vi "As PropertyObject.vi"(8 "error in (no error)":errorcluster, 11 "Execution in":refnum<class "Execution.lvclass">) -> (0 "error out":errorcluster, 2 "PropertyObject":refnum<k7>, 3 "Execution out":refnum<class "Execution.lvclass">)   [LabVIEW 2020, in "TSnax.lvlib" / "Execution.lvclass"]
uses:
  Execution.lvclass
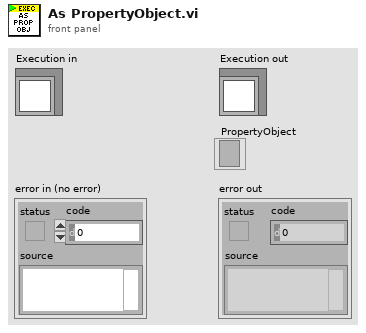
[diagram p1: front panel]
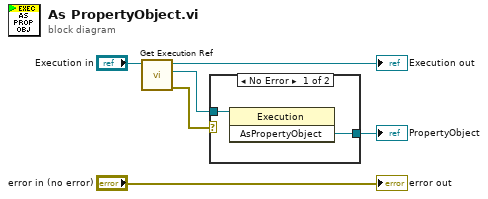
[diagram p0: block diagram]
diagram:
  n1 = call "Get Execution Ref.vi"("Execution in"="Execution in") -> ("error out"=w4:errorcluster, "Execution Ref"=w3:refnum<k7>, "Execution out"=→"Execution out":refnum<class "Execution.lvclass">)  [unwired: 8 in]
  n2 = case shown="No Error" w4 {
    tunnel: w3 -> [w8 _]
    tunnel: [w7 _] -> w2
    frame No Error {
      n3 = invoke class="Execution" method="AsPropertyObject"(reference=w8) -> ("AsPropertyObject"=w7:refnum<k7>)  [unwired: 2 in, 2 out]
    }
    frame Error {
    }
  }
  "PropertyObject" <- w2
  "error out" <- "error in (no error)"
